vi "Error Log Example.vi"() -> ()   [LabVIEW 2017]
uses:
  src/Serializer/Type Defs/Display Format.ctl
  src/Handler.UserEvent.Console/Handler.UserEvent.Console.lvclass
  \\192.168.1.40\Neosoft/Partage/Dossiers Personnels/BRO/DevTools_BR/wc/ErrorLog/src/Handler/Handler.lvclass
  src/Handler.File.Text/Handler.File.Text.lvclass
  src/Logger/Logger.lvclass
  src/Serializer/Serializer.lvlib
panel:
  in  "Name":string(combo)
  in  "Logger Display Format":T1=enum."PlainText.INI"
  in  "Logger Name":string="Logger Example"
  in  "Erase":bool
  in  "Show Console":bool
  in  "Error Level":T2(ring)
  in  "Error Message":string="Error log message."
  in  "Error":errorcluster={"status"=TRUE, "code"=5000, "source"="My Error Code"}
  in  "Send Error":bool
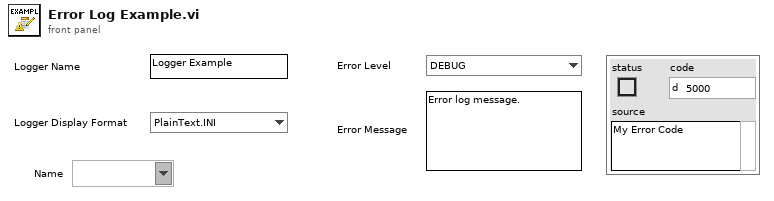
[diagram p1: front panel]
types:
  T1 = typedef "Serializer.lvlib/Display Format.ctl" = enum16{"PlainText", "PlainText.INI", "XML", "JSON"}
  T2 = enum16{"DEBUG", "INFO", "WARNING", "ERROR", "CRITICAL"}
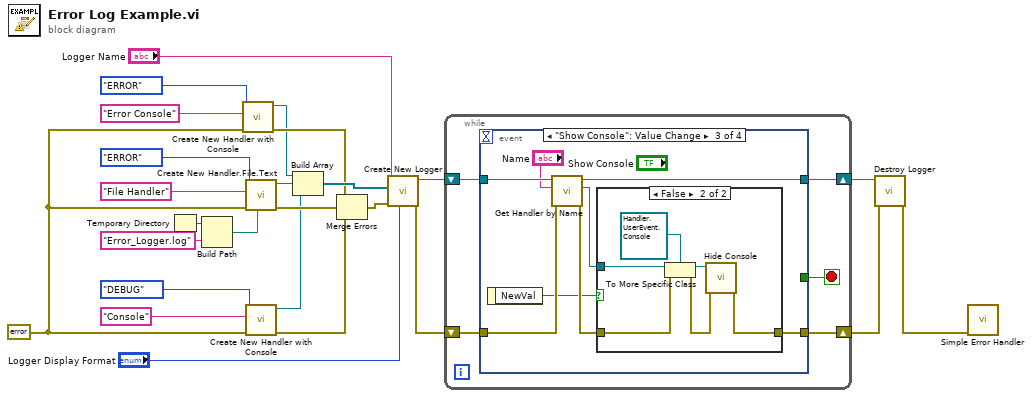
[diagram p0: block diagram]
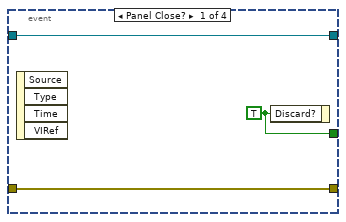
[diagram p2: hidden frame]
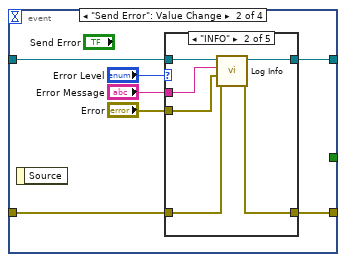
[diagram p3: hidden frame]
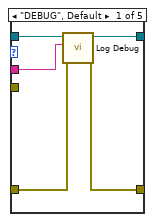
[diagram p4: hidden frame]
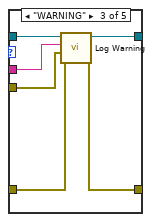
[diagram p5: hidden frame]
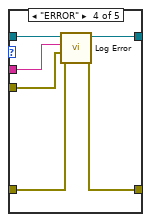
[diagram p6: hidden frame]
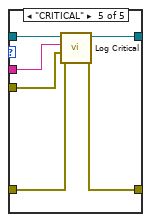
[diagram p7: hidden frame]
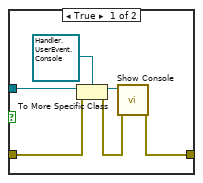
[diagram p8: hidden frame]
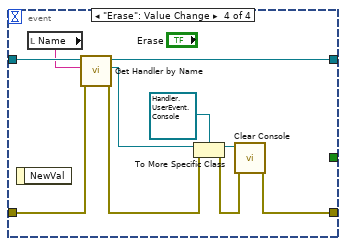
[diagram p9: hidden frame]
diagram:
  w5 = errorcluster {"status"=FALSE, "code"=0, "source"=""} ("error in (no error)")
  n1 = Temporary Directory() -> (w16:path)
  n2 = Build Path(base path=w16, name or relative path="Error_Logger.log") -> (appended path=w14:path)
  n3 = call "Create New Handler with Console.vi"("error in (no error)"=w5, "Name"="Error Console", "Level"=T2."ERROR") -> ("error out"=w4:errorcluster, "Handler.UserEvent.Console out"=w1:refnum<class "Handler.UserEvent.Console.lvclass">)  [unwired: 7 in]
  n4 = call "Create New Handler.File.Text.vi"("File Path"=w14, "error in (no error)"=w5, "Name"="File Handler", "Level"=T2."ERROR") -> ("error out"=w25:errorcluster, "Handler.File.Text out"=w24:refnum<class "Handler.File.Text.lvclass">)  [unwired: 6 in]
  n5 = call "Create New Handler with Console.vi"("error in (no error)"=w5, "Name"="Console", "Level"=T2."DEBUG") -> ("error out"=w12:errorcluster, "Handler.UserEvent.Console out"=w23:refnum<class "Handler.UserEvent.Console.lvclass">)  [unwired: 7 in]
  n6 = Build Array(w1, w24, w23) -> (w22:refnum<class "Handler.lvclass">[])
  n7 = Merge Errors(w4, w25, w12) -> (w21:errorcluster)
  n8 = call "Create New Logger.vi"("Display Format"="Logger Display Format", "error in (no error)"=w21, "Handlers"=w22, "Name"="Logger Name") -> ("error out"=w11:errorcluster, "Logger out"=w13:refnum<class "Logger.lvclass">)  [unwired: 6 in]
  n9 = while {
    shift-right: [w28] -> w10
    shift-left: w13 -> [w29]
    shift-right: [w26] -> w9
    shift-left: w11 -> [w27]
    stop <- w30 stop-if-true
    n10 = event shown="[2] \"Show Console\": Value Change" {
      selector: _ -> [_ _ _ _]
      dyn-events: _ -> [_ _ _ _]
      timeout: _ -> [_ _ _ _]
      tunnel: [w33 _ _ _] -> w30
      tunnel: w29 -> [w32 w40 w77 w99]
      tunnel: [w32 w39 w76 w98] -> w28
      tunnel: w27 -> [w31 w37 w75 w97]
      tunnel: [w31 w36 w72 w94] -> w26
      event Panel Close? {
        w33 = TRUE ("Discard?")
        n11 = event-data() -> ()  [unwired: 1 in, 4 out]
        n12 = event-data("Discard?"=w33) -> ()  [unwired: 1 in, 1 out]
      }
      event "Send Error": Value Change {
        n13 = event-data() -> ()  [unwired: 1 in, 1 out]
        n14 = case shown="\"INFO\"" "Error Level" {
          tunnel: w40 -> [w45 w51 w57 w63 w69]
          tunnel: [w44 w50 w56 w62 w68] -> w39
          tunnel: w37 -> [w43 w49 w55 w61 w67]
          tunnel: [w42 w48 w54 w60 w66] -> w36
          tunnel: "Error Message" -> [w41 w47 w53 w59 w65]
          tunnel: "Error" -> [_ w46 w52 w58 w64]
          frame "DEBUG", Default {
            n15 = call "Log Debug.vi"("error in (no error)"=w43, "Message"=w41, "Logger in"=w45) -> ("error out"=w42:errorcluster, "Logger out"=w44:refnum<class "Logger.lvclass">)  [unwired: 7 in]
          }
          frame "INFO" {
            n16 = call "Log Info.vi"("error in (no error)"=w49, "error"=w46, "Message"=w47, "Logger in"=w51) -> ("error out"=w48:errorcluster, "Logger out"=w50:refnum<class "Logger.lvclass">)  [unwired: 6 in]
          }
          frame "WARNING" {
            n17 = call "Log Warning.vi"("error in (no error)"=w55, "error"=w52, "Message"=w53, "Logger in"=w57) -> ("error out"=w54:errorcluster, "Logger out"=w56:refnum<class "Logger.lvclass">)  [unwired: 6 in]
          }
          frame "ERROR" {
            n18 = call "Log Error.vi"("error in (no error)"=w61, "error"=w58, "Message"=w59, "Logger in"=w63) -> ("error out"=w60:errorcluster, "Logger out"=w62:refnum<class "Logger.lvclass">)  [unwired: 6 in]
          }
          frame "CRITICAL" {
            n19 = call "Log Critical.vi"("error in (no error)"=w67, "error"=w64, "Message"=w65, "Logger in"=w69) -> ("error out"=w66:errorcluster, "Logger out"=w68:refnum<class "Logger.lvclass">)  [unwired: 6 in]
          }
        }
      }
      event "Show Console": Value Change {
        n20 = event-data() -> ("NewVal"=w71:bool)  [unwired: 1 in]
        n21 = call "Get Handler by Name.vi"("error in (no error)"=w75, "Handler Name"="Name", "Logger in"=w77) -> ("error out"=w73:errorcluster, "Handler"=w74:refnum<class "Handler.lvclass">, "Logger out"=w76:refnum<class "Logger.lvclass">)  [unwired: 6 in]
        n22 = case shown="False" w71 {
          tunnel: w74 -> [w83 w89]
          tunnel: w73 -> [w80 w86]
          tunnel: [w78 w84] -> w72
          frame True {
            n23 = To More Specific Class(target class=refnum<class "Handler.UserEvent.Console.lvclass"> refnum ("Error Log.lvlib:Handler.UserEvent.Console.lvclass"), reference=w83, error in=w80) -> (specific class reference=w82:refnum<class "Handler.UserEvent.Console.lvclass">, error out=w79:errorcluster)
            n24 = call "Show Console.vi"("error in (no error)"=w79, "Handler.UserEvent.Console in"=w82) -> ("error out"=w78:errorcluster)  [unwired: 8 in, 1 out]
          }
          frame False {
            n25 = To More Specific Class(target class=refnum<class "Handler.UserEvent.Console.lvclass"> refnum ("Error Log.lvlib:Handler.UserEvent.Console.lvclass"), reference=w89, error in=w86) -> (specific class reference=w88:refnum<class "Handler.UserEvent.Console.lvclass">, error out=w85:errorcluster)
            n26 = call "Hide Console.vi"("error in (no error)"=w85, "Handler.UserEvent.Console in"=w88) -> ("error out"=w84:errorcluster)  [unwired: 8 in, 1 out]
          }
        }
      }
      event "Erase": Value Change {
        n27 = event-data() -> ()  [unwired: 1 in, 1 out]
        n28 = local read "Name"() -> (w90:string)
        n29 = call "Get Handler by Name.vi"("error in (no error)"=w97, "Handler Name"=w90, "Logger in"=w99) -> ("error out"=w95:errorcluster, "Handler"=w96:refnum<class "Handler.lvclass">, "Logger out"=w98:refnum<class "Logger.lvclass">)  [unwired: 6 in]
        n30 = To More Specific Class(target class=refnum<class "Handler.UserEvent.Console.lvclass"> refnum ("Error Log.lvlib:Handler.UserEvent.Console.lvclass"), reference=w96, error in=w95) -> (specific class reference=w93:refnum<class "Handler.UserEvent.Console.lvclass">, error out=w91:errorcluster)
        n31 = call "Clear Console.vi"("error in (no error)"=w91, "Handler.UserEvent.Console in"=w93) -> ("error out"=w94:errorcluster)  [unwired: 8 in, 1 out]
      }
    }
  }
  n32 = call "Destroy Logger.vi"("error in (no error)"=w9, "Logger in"=w10) -> ("error out"=w8:errorcluster)  [unwired: 8 in, 1 out]
  n33 = call <vilib>:"Simple Error Handler.vi"("error in (no error)"=w8) -> ()  [unwired: 4 in, 5 out]
